vi "_PC_Daemon_TurboPump_Alone.vi"(8 "error in (no error)":errorcluster) -> (0 "error out":errorcluster)   [LabVIEW 2018]
uses:
  <vilib>/event_ctls.llb/eventvkey.ctl
  Library/RS485_TurboPump/clt/_ctl_PC_function_TC110.ctl
  PublicSubVI/Class/QMH/QMH.lvclass
panel:
  out "Turbo Status":string
  in  "rotating_speed":dbl=50.0 caption="rot.speed (%)"
  in  "SinpleMode.Pump On":bool
  in  "TC110 Settings":T1
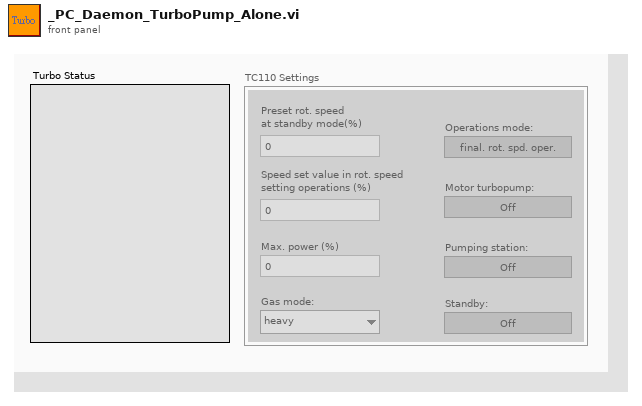
[diagram p1: front panel]
types:
  T1 = cluster{"Preset rot. speed \nat standby mode(%)":dbl, "Speed set value in rot. speed \nsetting operations (%)":dbl, "Max. power (%)":dbl, "Gas mode: ":enum16{"heavy", "light", "helium"}, "Operations mode: ":bool, "Motor turbopump: ":bool, "Pumping station: ":bool, "Standby: ":bool}
  T2 = enum8{"Enabled", "Disabled", "Disabled and Grayed Out"}
  T3 = typedef "eventvkey.ctl" = enum16{"ASCII", "Enter", "Return", "Shift", "Ctrl", "Alt", "Cmd", "Opt", "Caps", "NumLock", "Clear", "Break", "Up", "Down", "Left", "Right", "Insert", "Delete", "Home", "End", "PageUp", "PageDown", "Escape", "Help", "Pause", "ScrollLock", "F1", "F2", "F3", "F4", "F5", "F6", "F7", "F8", "F9", "F10", "F11", "F12", "F13", "F14", "F15", "F16", "F17", "F18", "F19", "F20", "F21", "F22", "F23", "F24", "Play", "VolumeUp", "VolumeDown", "Mute", "Two Byte Char"}
  T4 = typedef "_ctl_PC_function_TC110.ctl" = enum16{"Initialisation", "Read status", "Write command", "Read command", "Close"}
  T5 = typedef "_ctl_PC_TurboSettings.ctl" = cluster{"Preset rot. speed \nat standby mode(%)":dbl, "Speed set value in rot. speed \nsetting operations (%)":dbl, "Max. power (%)":dbl, "Gas mode: ":enum16{"heavy", "light", "helium"}, "Operations mode: ":bool, "Motor turbopump: ":bool, "Pumping station: ":bool, "Standby: ":bool}
  T6 = cluster{"Motor voltage":string, "Actual power":string, "Target speed":string, "Actual speed":string, "Temp. of electronics":string, "Temp. of pump bottom":string}
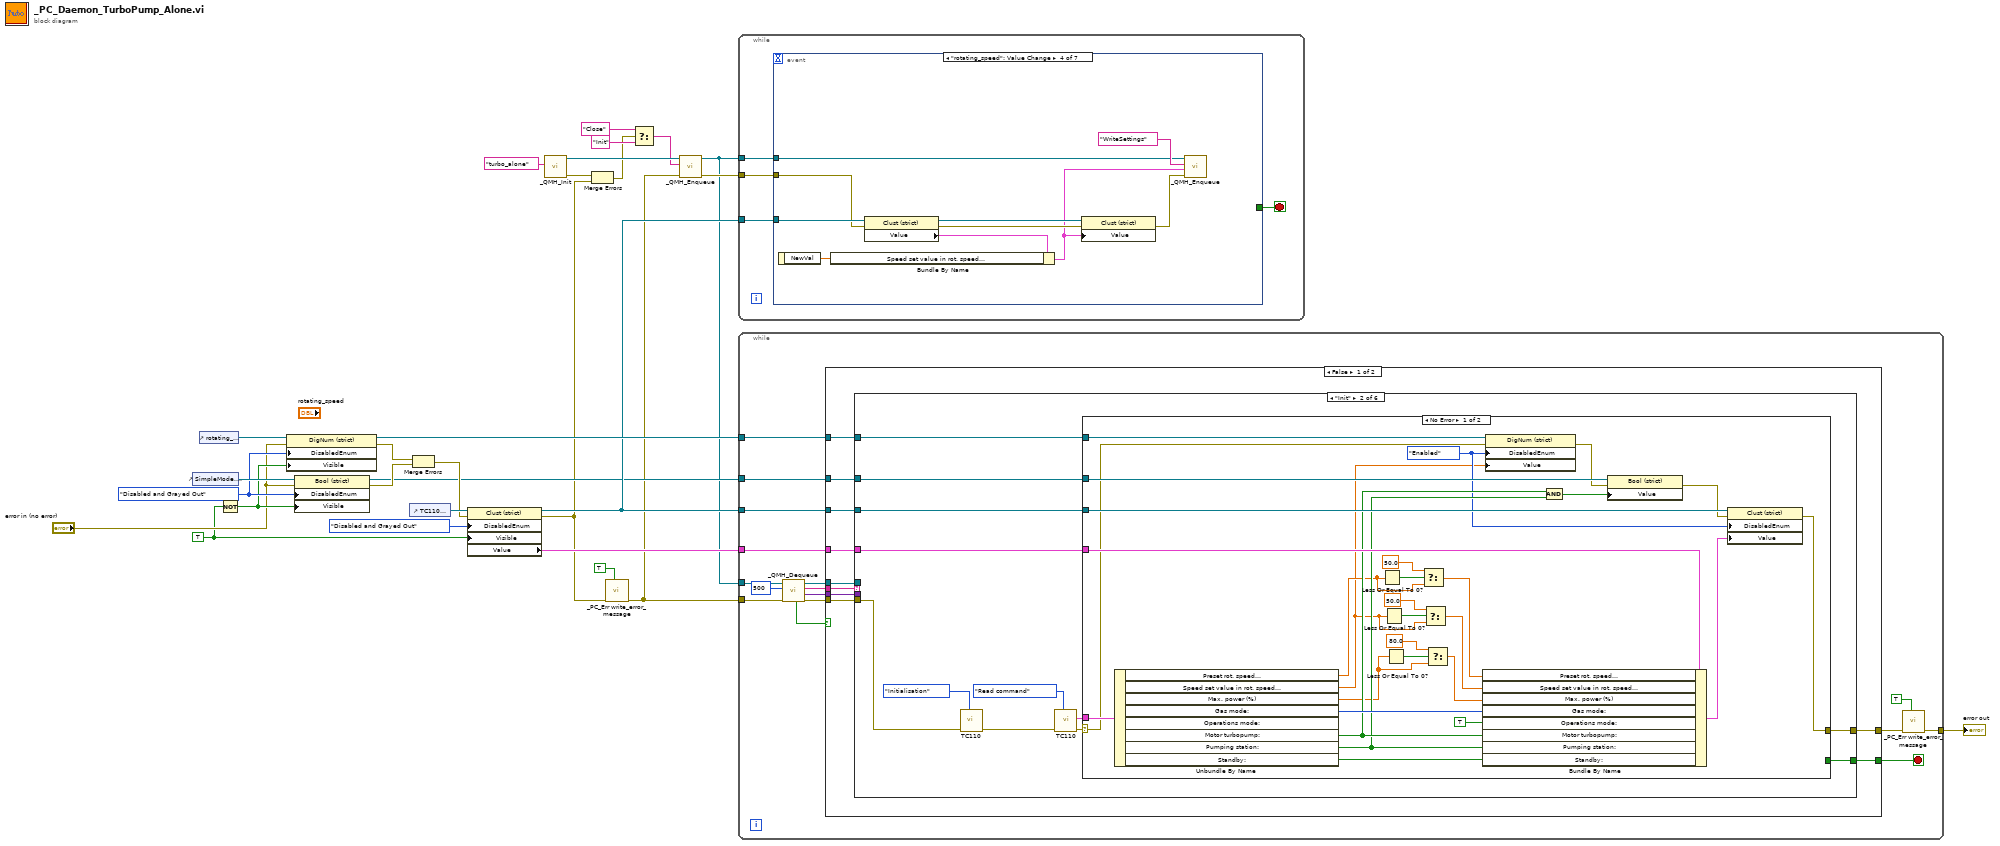
[diagram p0: block diagram]
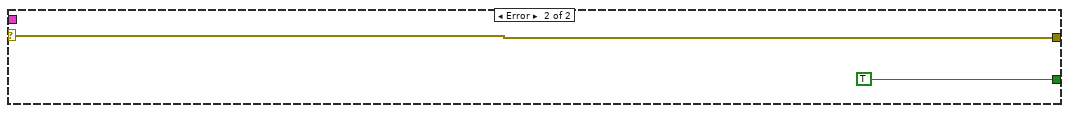
[diagram p3: hidden frame]
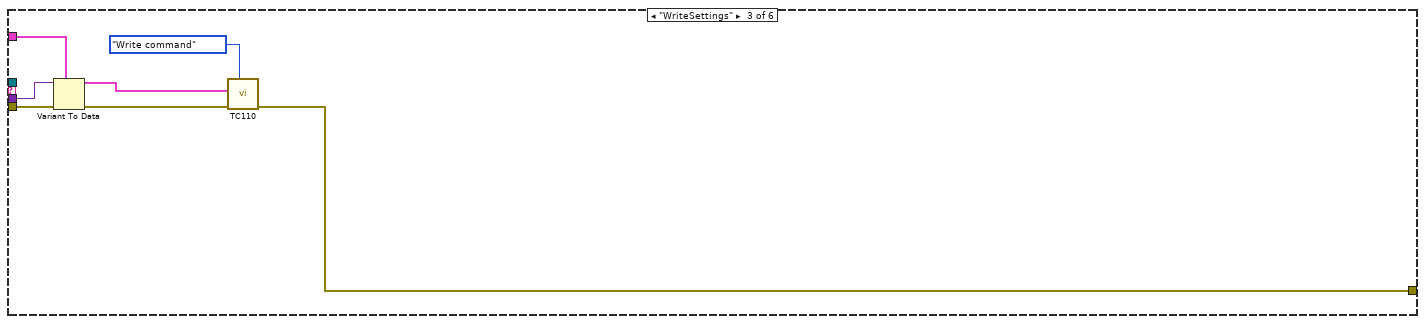
[diagram p4: hidden frame]
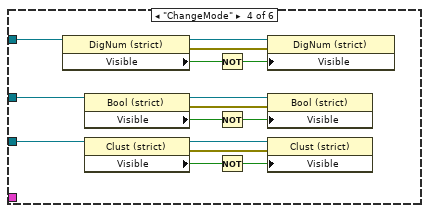
[diagram p5: hidden frame]
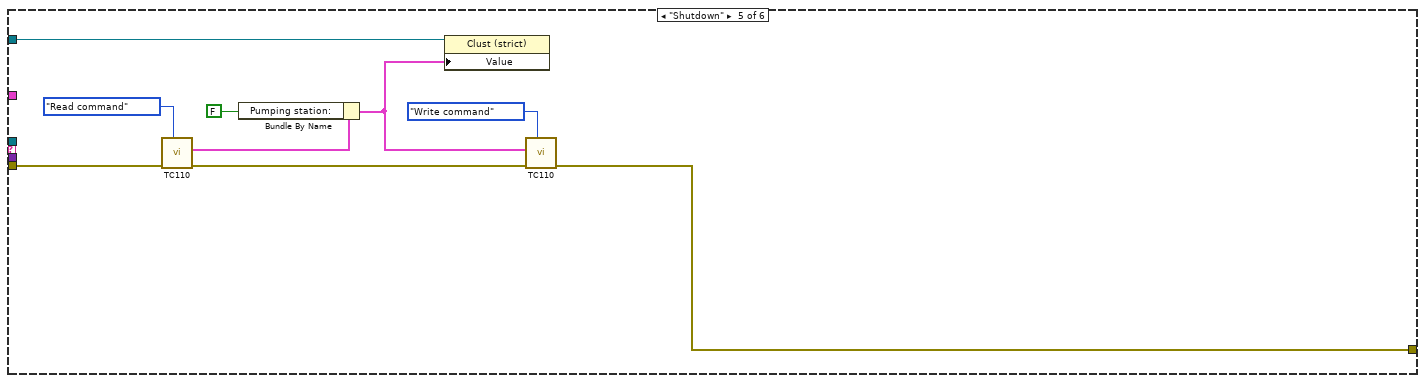
[diagram p6: hidden frame]
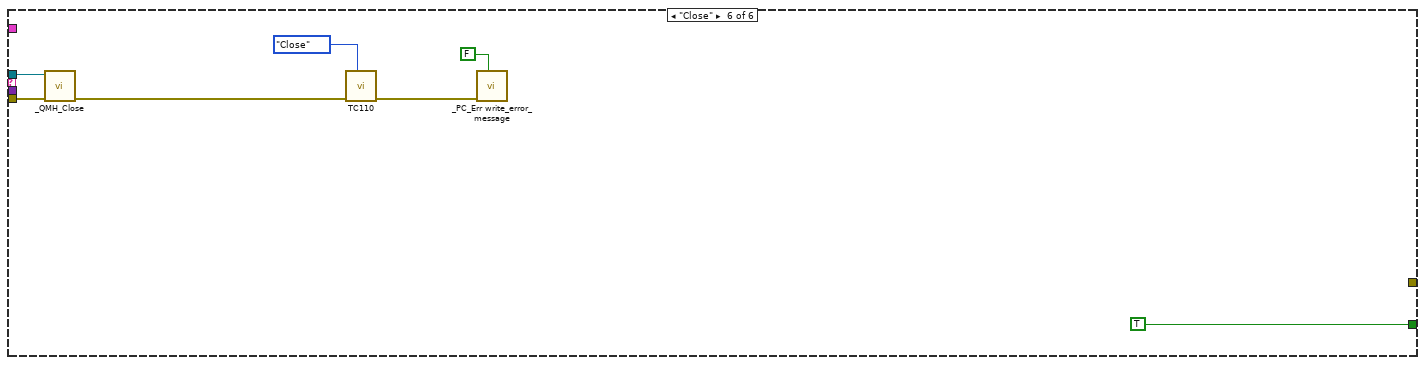
[diagram p7: hidden frame]
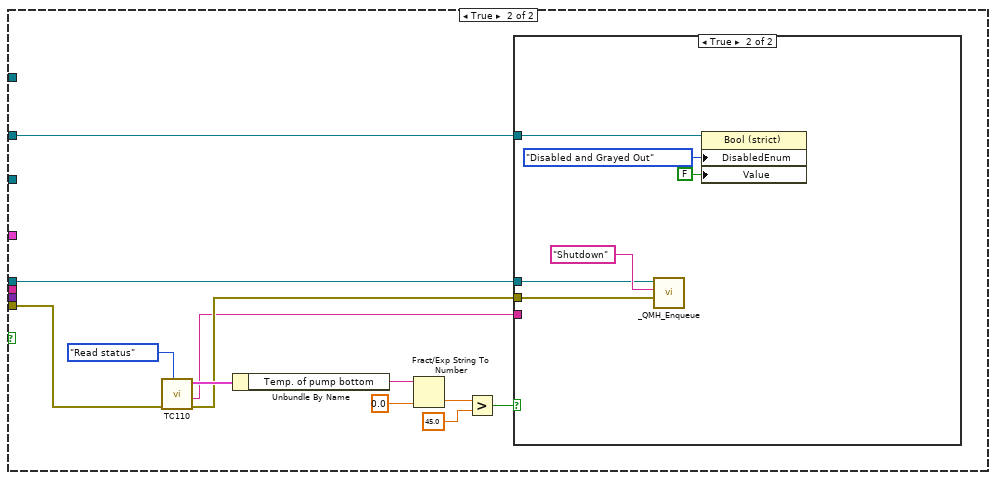
[diagram p8: hidden frame]
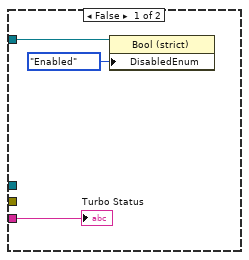
[diagram p9: hidden frame]
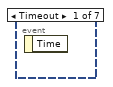
[diagram p10: hidden frame]
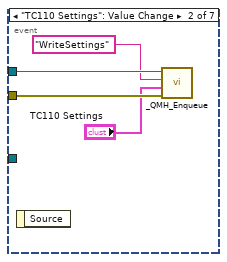
[diagram p11: hidden frame]
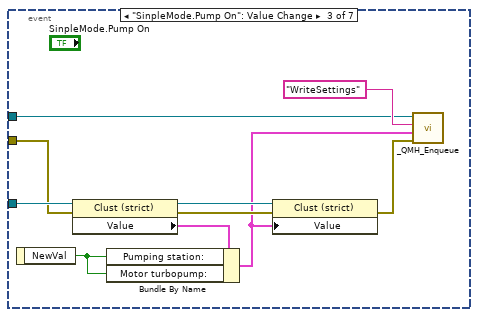
[diagram p12: hidden frame]
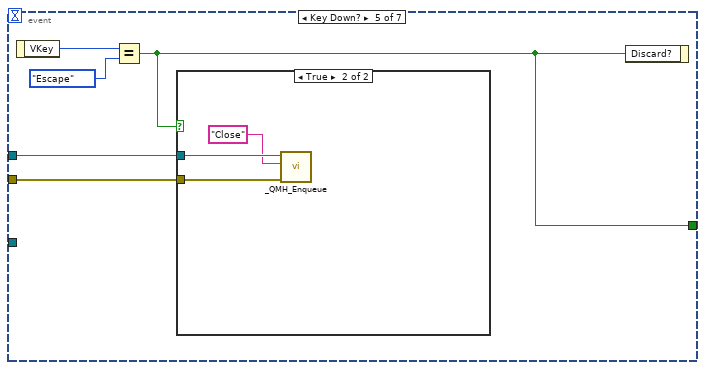
[diagram p13: hidden frame]
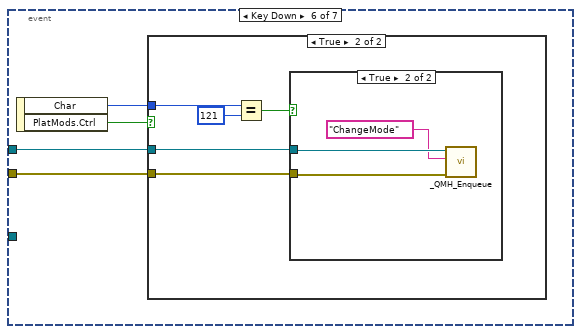
[diagram p15: hidden frame]
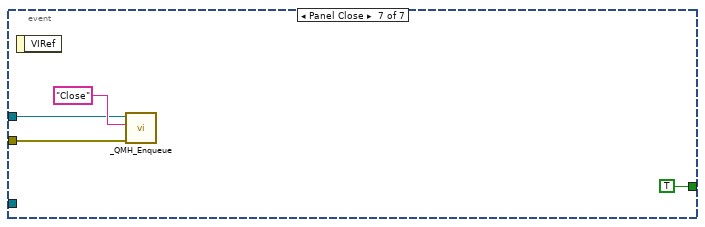
[diagram p18: hidden frame]
diagram:
  w1 = TRUE ("x")
  w23 = T2."Disabled and Grayed Out" ("Disabled")
  n1 = control-ref of="SimpleMode.Pump On"() -> (w25:refnum<vi>)
  n2 = control-ref of="rotating_speed"() -> (w21:refnum<vi>)
  n3 = Not(x=w1) -> (.not. x?=w22:bool)
  n4 = property class="DigNum (strict)"(reference=w21, error in="error in (no error)", "DisabledEnum"=w23, "Visible"=w22) -> (reference out=w14:refnum<vi>, error out=w18:errorcluster)
  n5 = property class="Bool (strict)"(reference=w25, error in="error in (no error)", "DisabledEnum"=w23, "Visible"=w22) -> (reference out=w12:refnum<vi>, error out=w17:errorcluster)
  n6 = control-ref of="TC110 Settings"() -> (w28:refnum<vi>)
  n7 = Merge Errors(w18, w17) -> (w16:errorcluster)
  n8 = property class="Clust (strict)"(reference=w28, error in=w16, "DisabledEnum"=T2."Disabled and Grayed Out" ("Disabled"), "Visible"=w1) -> (reference out=w13:refnum<vi>, error out=w6:errorcluster, "Value"=w26:T1)
  n9 = call "_QMH_Init.vi"("name (unnamed)"="turbo_alone") -> ("error out"=w7:errorcluster, "QMH out"=w10:refnum<class "QMH.lvclass">)  [unwired: 9 in]
  n10 = Merge Errors(w7, w6) -> (w5:errorcluster)
  n11 = call "_PC_Err write_error_message.vi"("show msg( T )"=TRUE, "error in"=w6) -> ("error out"=w4:errorcluster)  [unwired: 9 in]
  n12 = Select(t="Close" ("Msg"), s=w5, f="Init" ("Msg")) -> (s? t:f=w9:string)
  n13 = call "_QMH_Enqueue.vi"("error in (no error)"=w4, "Msg"=w9, "QMH in"=w10) -> ("error out"=w8:errorcluster, "QMH out"=w3:refnum<class "QMH.lvclass">)  [unwired: 7 in]
  n14 = while {
    tunnel: w13 -> [w31]
    tunnel: w8 -> [w30]
    tunnel: w3 -> [w29]
    stop <- w32 stop-if-true
    n15 = event shown="[3] \"rotating_speed\": Value Change" {
      selector: _ -> [_ _ _ _ _ _ _]
      dyn-events: _ -> [_ _ _ _ _ _ _]
      timeout: _ -> [_ _ _ _ _ _ _]
      tunnel: [_ _ _ _ w59 _ TRUE] -> w32
      tunnel: w31 -> [_ _ w45 w56 _ _ _]
      tunnel: w30 -> [_ w35 w38 w48 w57 w65 w77]
      tunnel: w29 -> [_ w36 w39 w49 w58 w66 w78]
      event Timeout {
        n16 = event-data() -> ()  [unwired: 1 in, 1 out]
      }
      event "TC110 Settings": Value Change {
        n17 = event-data() -> ()  [unwired: 1 in, 1 out]
        n18 = call "_QMH_Enqueue.vi"("error in (no error)"=w35, "Data"="TC110 Settings", "Msg"="WriteSettings", "QMH in"=w36) -> ()  [unwired: 6 in, 2 out]
      }
      event "SinpleMode.Pump On": Value Change {
        n19 = event-data() -> ("NewVal"=w46:bool)  [unwired: 1 in]
        n20 = property class="Clust (strict)"(reference=w45, error in=w38) -> (reference out=w43:refnum<vi>, error out=w42:errorcluster, "Value"=w44:T1)
        n21 = Bundle By Name(cluster=w44, "Pumping station:"=w46, "Motor turbopump:"=w46) -> (w40:T1)
        n22 = property class="Clust (strict)"(reference=w43, error in=w42, "Value"=w40) -> (error out=w37:errorcluster)  [unwired: 1 out]
        n23 = call "_QMH_Enqueue.vi"("error in (no error)"=w37, "Data"=w40, "Msg"="WriteSettings", "QMH in"=w39) -> ()  [unwired: 6 in, 2 out]
      }
      event "rotating_speed": Value Change {
        n24 = event-data() -> ("NewVal"=w52:dbl)  [unwired: 1 in]
        n25 = property class="Clust (strict)"(reference=w56, error in=w48) -> (reference out=w54:refnum<vi>, error out=w53:errorcluster, "Value"=w55:T1)
        n26 = Bundle By Name(cluster=w55, "Speed set value in rot. speed \nsetting operations (%)"=w52) -> (w47:T1)
        n27 = property class="Clust (strict)"(reference=w54, error in=w53, "Value"=w47) -> (error out=w50:errorcluster)  [unwired: 1 out]
        n28 = call "_QMH_Enqueue.vi"("error in (no error)"=w50, "Data"=w47, "Msg"="WriteSettings", "QMH in"=w49) -> ()  [unwired: 6 in, 2 out]
      }
      event Key Down? {
        n29 = event-data() -> ("VKey"=w61:T3)  [unwired: 1 in]
        n30 = Equal?(x=w61, y=eventvkey."Escape") -> (x = y?=w59:bool)
        n31 = case shown="True" w59 {
          tunnel: w58 -> [_ w64]
          tunnel: w57 -> [_ w63]
          frame False {
          }
          frame True {
            n32 = call "_QMH_Enqueue.vi"("error in (no error)"=w63, "Msg"="Close", "QMH in"=w64) -> ()  [unwired: 7 in, 2 out]
          }
        }
        n33 = event-data("Discard?"=w59) -> ()  [unwired: 1 in, 1 out]
      }
      event Key Down {
        n34 = event-data() -> ("Char"=w67:i16, "PlatMods.Ctrl"=w68:bool)  [unwired: 1 in]
        n35 = case shown="True" w68 {
          tunnel: w67 -> [_ w73]
          tunnel: w66 -> [_ w70]
          tunnel: w65 -> [_ w71]
          frame False {
          }
          frame True {
            n36 = Equal?(x=w73, y=i16 121) -> (x = y?=w69:bool)
            n37 = case shown="True" w69 {
              tunnel: w71 -> [_ w76]
              tunnel: w70 -> [_ w75]
              frame False {
              }
              frame True {
                n38 = call "_QMH_Enqueue.vi"("error in (no error)"=w76, "Msg"="ChangeMode", "QMH in"=w75) -> ()  [unwired: 7 in, 2 out]
              }
            }
          }
        }
      }
      event Panel Close {
        n39 = event-data() -> ()  [unwired: 1 in, 1 out]
        n40 = call "_QMH_Enqueue.vi"("error in (no error)"=w77, "Msg"="Close", "QMH in"=w78) -> ()  [unwired: 7 in, 2 out]
      }
    }
  }
  n41 = while {
    tunnel: w26 -> [w96]
    tunnel: w13 -> [w95]
    tunnel: w12 -> [w94]
    tunnel: [w92] -> w24
    tunnel: w14 -> [w90]
    tunnel: w4 -> [w88]
    tunnel: w3 -> [w87]
    stop <- w89 stop-if-true
    n42 = call "_QMH_Dequeue.vi"("error in (no error)"=w88, "timeout in ms (-1)"=500, "QMH in"=w87) -> ("error out"=w84:errorcluster, "Data"=w83:variant, "Msg"=w82:string, "QMH out"=w81:refnum<class "QMH.lvclass">, "timed out?"=w85:bool)  [unwired: 3 in, 1 out]
    n43 = case shown="False" w85 {
      tunnel: w96 -> [w106 _]
      tunnel: w95 -> [w105 _]
      tunnel: w94 -> [w104 w188]
      tunnel: [w103 _] -> w91
      tunnel: [w102 _] -> w89
      tunnel: w90 -> [w101 _]
      tunnel: w84 -> [w99 w198]
      tunnel: w83 -> [w98 _]
      tunnel: w82 -> [w100 _]
      tunnel: w81 -> [w97 w191]
      frame False {
        n44 = case shown="\"Init\"" w100 {
          tunnel: [_ w107 _ _ _ TRUE] -> w102
          tunnel: w106 -> [_ w118 w152 _ _ _]
          tunnel: w105 -> [_ w117 _ w170 w173 _]
          tunnel: w104 -> [_ w116 _ w171 _ _]
          tunnel: [_ w115 w150 _ w174 _] -> w103
          tunnel: w101 -> [_ w114 _ w169 _ _]
          tunnel: w99 -> [_ w109 w155 _ w175 w185]
          tunnel: w98 -> [_ _ w156 _ _ _]
          tunnel: w97 -> [_ _ _ _ _ w186]
          frame Default {
          }
          frame "Init" {
            n45 = call "TC110.vi"("Function"=_ctl_PC_function_TC110."Initialisation", "Error in"=w109) -> ("Error out"=w111:errorcluster)  [unwired: 6 in, 3 out]
            n46 = call "TC110.vi"("Function"=_ctl_PC_function_TC110."Read command", "Error in"=w111) -> ("Error out"=w108:errorcluster, "Settings out"=w110:T5)  [unwired: 6 in, 2 out]
            n47 = case shown="No Error" w108 {
              selector: w108 -> [w132 w149]
              tunnel: w118 -> [w147 _]
              tunnel: w117 -> [w146 _]
              tunnel: w116 -> [w145 _]
              tunnel: [w144 w149] -> w115
              tunnel: w114 -> [w143 _]
              tunnel: w110 -> [w133 _]
              tunnel: [_ TRUE] -> w107
              frame No Error {
                w136 = T2."Enabled" ("Disabled")
                n48 = Unbundle By Name(w133) -> ("Preset rot. speed \nat standby mode(%)"=w129:dbl, "Speed set value in rot. speed \nsetting operations (%)"=w123:dbl, "Max. power (%)"=w122:dbl, "Gas mode:"=w142:enum16{"heavy", "light", "helium"}, "Motor turbopump:"=w139:bool, "Pumping station:"=w138:bool, "Standby:"=w141:bool)  [unwired: 1 out]
                n49 = Less Or Equal To 0?(x=w129) -> (x <= 0?=w130:bool)
                n50 = Less Or Equal To 0?(x=w123) -> (x <= 0?=w127:bool)
                n51 = Less Or Equal To 0?(x=w122) -> (x <= 0?=w125:bool)
                n52 = Select(t=50.0, s=w130, f=w129) -> (s? t:f=w119:dbl)
                n53 = Select(t=50.0, s=w127, f=w123) -> (s? t:f=w120:dbl)
                n54 = Select(t=80.0, s=w125, f=w122) -> (s? t:f=w121:dbl)
                n55 = Bundle By Name(cluster=w147, "Preset rot. speed \nat standby mode(%)"=w119, "Speed set value in rot. speed \nsetting operations (%)"=w120, "Max. power (%)"=w121, "Gas mode:"=w142, "Operations mode:"=TRUE, "Motor turbopump:"=w139, "Pumping station:"=w138, "Standby:"=w141) -> (w140:T1)
                n56 = property class="DigNum (strict)"(reference=w143, error in=w132, "DisabledEnum"=w136, "Value"=w123) -> (error out=w135:errorcluster)  [unwired: 1 out]
                n57 = And(x=w139, y=w138) -> (x .and. y?=w137:bool)
                n58 = property class="Bool (strict)"(reference=w145, error in=w135, "Value"=w137) -> (error out=w134:errorcluster)  [unwired: 1 out]
                n59 = property class="Clust (strict)"(reference=w146, error in=w134, "DisabledEnum"=w136, "Value"=w140) -> (error out=w144:errorcluster)  [unwired: 1 out]
              }
              frame Error {
              }
            }
          }
          frame "WriteSettings" {
            n60 = Variant To Data(error in=w155, type=w152, Variant=w156) -> (data=w151:T1, error out=w153:errorcluster)
            n61 = call "TC110.vi"("Function"=_ctl_PC_function_TC110."Write command", "Error in"=w153, "Settings in"=w151) -> ("Error out"=w150:errorcluster)  [unwired: 5 in, 3 out]
          }
          frame "ChangeMode" {
            n62 = property class="DigNum (strict)"(reference=w169) -> (reference out=w168:refnum<vi>, error out=w167:errorcluster, "Visible"=w158:bool)  [unwired: 1 in]
            n63 = property class="Bool (strict)"(reference=w171) -> (reference out=w166:refnum<vi>, error out=w165:errorcluster, "Visible"=w160:bool)  [unwired: 1 in]
            n64 = property class="Clust (strict)"(reference=w170) -> (reference out=w164:refnum<vi>, error out=w163:errorcluster, "Visible"=w162:bool)  [unwired: 1 in]
            n65 = Not(x=w158) -> (.not. x?=w157:bool)
            n66 = Not(x=w160) -> (.not. x?=w159:bool)
            n67 = Not(x=w162) -> (.not. x?=w161:bool)
            n68 = property class="DigNum (strict)"(reference=w168, error in=w167, "Visible"=w157) -> ()  [unwired: 2 out]
            n69 = property class="Bool (strict)"(reference=w166, error in=w165, "Visible"=w159) -> ()  [unwired: 2 out]
            n70 = property class="Clust (strict)"(reference=w164, error in=w163, "Visible"=w161) -> ()  [unwired: 2 out]
          }
          frame "Shutdown" {
            n71 = call "TC110.vi"("Function"=_ctl_PC_function_TC110."Read command", "Error in"=w175) -> ("Error out"=w176:errorcluster, "Settings out"=w177:T5)  [unwired: 6 in, 2 out]
            n72 = Bundle By Name(cluster=w177, "Pumping station:"=FALSE) -> (w172:T5)
            n73 = property class="Clust (strict)"(reference=w173, "Value"=w172) -> ()  [unwired: 1 in, 2 out]
            n74 = call "TC110.vi"("Function"=_ctl_PC_function_TC110."Write command", "Error in"=w176, "Settings in"=w172) -> ("Error out"=w174:errorcluster)  [unwired: 5 in, 3 out]
          }
          frame "Close" {
            n75 = call "_QMH_Close.vi"("error in (no error)"=w185, "QMH in"=w186) -> ("error out"=w183:errorcluster)  [unwired: 9 in]
            n76 = call "TC110.vi"("Function"=_ctl_PC_function_TC110."Close", "Error in"=w183) -> ("Error out"=w181:errorcluster)  [unwired: 6 in, 3 out]
            n77 = call "_PC_Err write_error_message.vi"("show msg( T )"=FALSE, "error in"=w181) -> ()  [unwired: 9 in, 1 out]
          }
        }
      }
      frame True {
        n78 = call "TC110.vi"("Function"=_ctl_PC_function_TC110."Read status", "Error in"=w198) -> ("Error out"=w190:errorcluster, "Status_string"=w189:string, "output cluster"=w196:T6)  [unwired: 6 in, 1 out]
        n79 = Unbundle By Name(w196) -> ("Temp. of pump bottom"=w195:string)
        n80 = Fract/Exp String To Number(string=w195, default (0 dbl)=sgl 0.0 ("default (0 DBL)")) -> (number=w193:sgl)  [unwired: 2 in, 1 out]
        n81 = Greater?(x=w193, y=sgl 45.0) -> (0:w192:bool)
        n82 = case shown="True" w192 {
          tunnel: w191 -> [_ w207]
          tunnel: w190 -> [_ w206]
          tunnel: w189 -> [w202 _]
          tunnel: w188 -> [w201 w205]
          frame False {
            n83 = property class="Bool (strict)"(reference=w201, "DisabledEnum"=T2."Enabled" ("Disabled")) -> ()  [unwired: 1 in, 2 out]
            "Turbo Status" <- w202
          }
          frame True {
            n84 = call "_QMH_Enqueue.vi"("Data"=w206, "Msg"="Shutdown", "QMH in"=w207) -> ()  [unwired: 7 in, 2 out]
            n85 = property class="Bool (strict)"(reference=w205, "DisabledEnum"=T2."Disabled and Grayed Out" ("Disabled"), "Value"=FALSE) -> ()  [unwired: 1 in, 2 out]
          }
        }
      }
    }
    n86 = call "_PC_Err write_error_message.vi"("show msg( T )"=TRUE, "error in"=w91) -> ("error out"=w92:errorcluster)  [unwired: 9 in]
  }
  "error out" <- w24
